vi "Read Buffer Statistic.vi"(7 "Statistic (0: Mean)":u16(ring) items=["Mean", "Standard Deviation", "Maximum", "Minimum"], 8 "error in":errorcluster, 11 "VISA resource name":refnum<visa-resource-name>) -> (0 "error out":errorcluster, 2 "Statistic Value":dbl, 3 "VISA resource name out":refnum<visa-resource-name>)   [LabVIEW 2020, in "Keithley 2182.lvlib"]
doc: "Fetches the specified statistic of the data buffer."
uses:
  Keithley 2182.lvlib
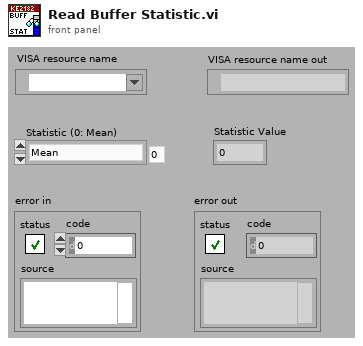
[diagram p1: front panel]
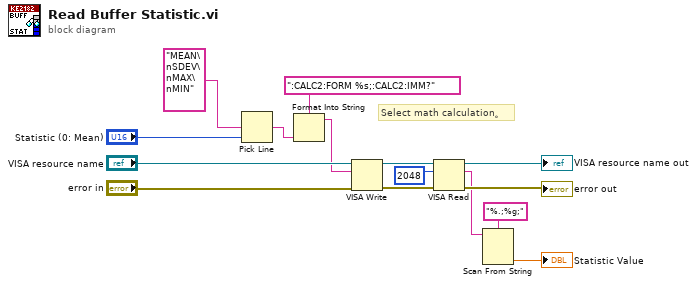
[diagram p0: block diagram]
diagram:
  # "Select math calculation。"
  n1 = Pick Line(multi-line string="MEAN\nSDEV\nMAX\nMIN", line index="Statistic (0: Mean)") -> (output string=w4:string)  [unwired: 1 in]
  n2 = Format Into String(format string=":CALC2:FORM %s;:CALC2:IMM?" ("string (\"\")"), w4) -> (resulting string=w1:string)  [unwired: 2 in, 1 out]
  n3 = VISA Write(VISA resource name="VISA resource name", write buffer=w1, error in (no error)="error in") -> (VISA resource name out=w14:refnum<visa-resource-name>, error out=w15:errorcluster)  [unwired: 1 out]
  n4 = VISA Read(VISA resource name=w14, byte count=u32 2048, error in (no error)=w15) -> (VISA resource name out=→"VISA resource name out":refnum<visa-resource-name>, read buffer=w10:string, error out=→"error out":errorcluster)  [unwired: 1 out]
  n5 = Scan From String(format string="%.;%g;", input string=w10) -> (output 1=→"Statistic Value":dbl)  [unwired: 3 in, 3 out]
